vi "OdometrySystem.vi"() -> ()   [LabVIEW 2025]
panel:
  out "IntakeSystem/IntakeMotorOut 3":dbl caption="Rotation Rad" format="%11.2f"
  out "IntakeSystem/IntakeMotorOut 2":dbl caption="Y Pos M" format="%11.2f"
  out "IntakeSystem/IntakeMotorRPM":dbl caption="Elapsed Time" format="%9.3f"
  out "IntakeSystem/IntakeMotorOut":dbl caption="X Pos M" format="%11.2f"
  # "ODOMETRY"
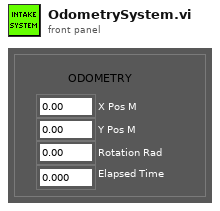
[diagram p1: front panel]
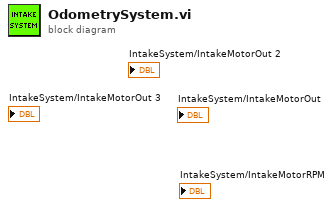
[diagram p0: block diagram]
diagram:
